vi "时间与数值的转换.vi"() -> ()   [LabVIEW 2023]
doc: "本VI是为《我和LabVIEW》一书编写的示例。\n关于本书的介绍请参考网页：\nhttp://ruanqizhen.spaces.live.com/blog/cns!5852D4F797C53FB6!4310.entry"
panel:
  out "手工转换整数部分":u64
  out "手工转换小数部分":ext format="%#.6f"
  out "内部类型":cluster{u64, u64} {"?" format="%016x"; "?" format="%016x"}
  out "直接转换得到的秒数":dbl format="%.6f"
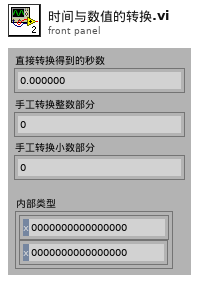
[diagram p1: front panel]
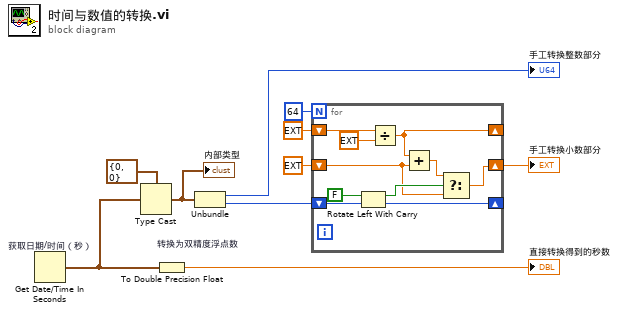
[diagram p0: block diagram]
diagram:
  n1 = Get Date/Time In Seconds "获取日期/时间（秒）"() -> (seconds since 1Jan1904=w10:timestamp)
  n2 = Type Cast(type=cluster{u64, u64} {0, 0}, x=w10) -> (*(type *) &x=w8:cluster{u64, u64})
  "内部类型" <- w8
  n3 = To Double Precision Float "转换为双精度浮点数"(number=w10) -> (double precision float=→"直接转换得到的秒数":dbl)
  n4 = Unbundle(w8) -> (→"手工转换整数部分":u64, w6:u64)
  n5 = for {
    N: 64 -> [_]
    shift-right: [w19] -> _
    shift-left: w6 -> [w20]
    shift-right: [w15] -> _
    shift-left: ext 1.0 -> [w18]
    shift-right: [w12] -> w4
    shift-left: ext 0.0 ("扩展精度浮点数") -> [w13]
    n6 = Rotate Left With Carry(2:w20, 3:FALSE ("进位")) -> (0:w19:u64, 1:w16:bool)
    n7 = Divide(x=w18, y=ext 2.0) -> (x/y=w15:ext)
    n8 = Add(x=w15, y=w13) -> (x+y=w14:ext)
    n9 = Select(t=w14, s=w16, f=w13) -> (s? t:f=w12:ext)
  }
  "手工转换小数部分" <- w4
